vi "QTrkGetQueueLength.vi"(8 "error in (no error)":errorcluster, 11 "QTrk Instance":T1) -> (0 "error out":errorcluster, 1 "maxQueueLen":i32, 2 "queue size":i32, 3 "QTrk Instance":T1)   [LabVIEW 2011]
uses:
  QTrkInstance.ctl
  QTrkDLL.vi
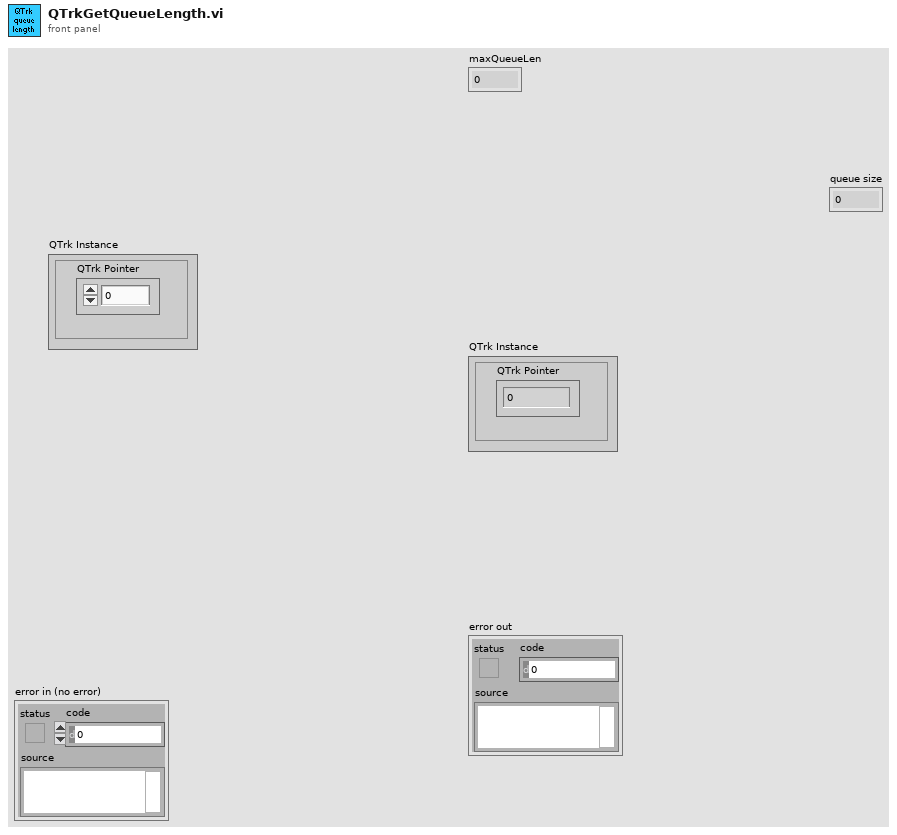
[diagram p1: front panel]
types:
  T1 = typedef "QTrkInstance.ctl" = cluster{"QTrk Pointer":u64}
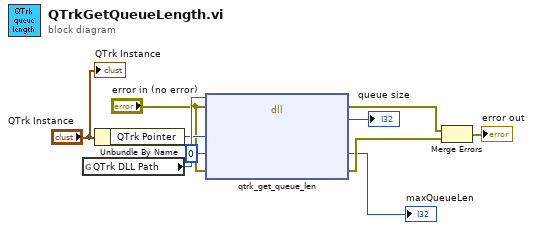
[diagram p0: block diagram]
diagram:
  n1 = global read "QTrkDLL.vi" "QTrk DLL Path"() -> (w9:path)
  n2 = Unbundle By Name("QTrk Instance") -> ("QTrk Pointer"=w8:u64)
  n3 = dll-call lib="D:/jcnossen1/cudaqi-tracker/bin/jtrk-labview.dll" fn="qtrk_get_queue_len"(path in=w9, error in="error in (no error)", "tracker"=w8, "maxQueueLen"=0, "error"="error in (no error)") -> (error out=w5:errorcluster, "return type"=→"queue size":i32, "maxQueueLen"=→"maxQueueLen":i32, "error"=w4:errorcluster)  [unwired: 2 in, 1 out]
  n4 = Merge Errors(w5, w4) -> (→"error out":errorcluster)
  "QTrk Instance" <- "QTrk Instance"
